vi "VCS Activate Position Mode.vi"(8 "error in (no error)":errorcluster, 11 "axis in":cluster{"keyHandle":u32, "nodeId":u16}={"keyHandle"=0, "nodeId"=1}) -> (0 "error out":errorcluster, 3 "axis out":cluster{"keyHandle":u32, "nodeId":u16}={"keyHandle"=0, "nodeId"=1})   [LabVIEW 2017, in "maxonEPOS.lvlib"]
doc: "With the function <B>VCS_ActivatePositionMode</B> the device changes to position mode (PM)."
uses:
  Examples/maxonEPOS.lvlib
  SSI_Tool/InstrumentsInterfaces/Motordriver/maxon EPOS/Resources/EposCmd.dll
  SSI_Tool/InstrumentsInterfaces/Motordriver/maxon EPOS/Resources/EposCmd64.dll
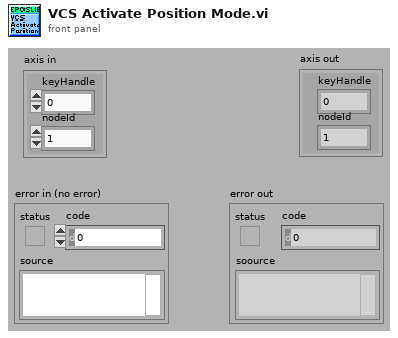
[diagram p1: front panel]
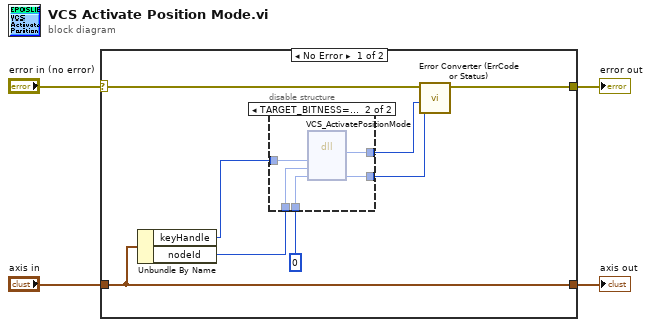
[diagram p0: block diagram]
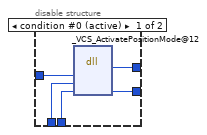
[diagram p2: hidden frame]
diagram:
  n1 = case shown="No Error" "error in (no error)" {
    selector: "error in (no error)" -> [w10 w23]
    tunnel: "axis in" -> [w12 w24]
    tunnel: [w12 w24] -> w3
    tunnel: [w11 w23] -> w2
    frame No Error {
      n2 = Unbundle By Name(w12) -> ("keyHandle"=w6:u32, "nodeId"=w5:u16)
      n3 = disable-structure shown="TARGET_BITNESS==64" {
        disable-tunnel: u32 0 ("pErrorCode") -> [w17 w22]
        disable-tunnel: [w16 w21] -> w8
        disable-tunnel: [w15 w20] -> w7
        disable-tunnel: w6 -> [w14 w19]
        disable-tunnel: w5 -> [w13 w18]
        frame condition #0 (active) {
          n4 = dll-call lib="C:/workspace/project/scancon/sw/SSI_Tool/InstrumentsInterfaces/Motordriver/maxon EPOS/Resources/EposCmd.*" fn="_VCS_ActivatePositionMode@12"("KeyHandle"=w14, "NodeId"=w13, "pErrorCode"=w17) -> (w15:i32, "pErrorCode"=w16:u32)  [unwired: 5 in, 2 out]
        }
        frame condition #1 {
          n5 = dll-call lib="C:/setup/Resources/EposCmd64.*" fn="VCS_ActivatePositionMode" ("EposCmd.dll:_VCS_ActivatePositionMode@12")("KeyHandle"=w19, "NodeId"=w18, "pErrorCode"=w22) -> ("Rückgabetyp"=w20:i32, "pErrorCode"=w21:u32)  [unwired: 5 in, 2 out]
        }
      }
      n6 = call "Error Converter (ErrCode or Status).vi"("error code"=w8, "return type"=w7, "error in (no error)"=w10) -> ("error out"=w11:errorcluster)  [unwired: 7 in]
    }
    frame Error {
    }
  }
  "error out" <- w2
  "axis out" <- w3
